vi "主函数.vi"() -> ()   [LabVIEW 2013]
uses:
  <vilib>/userdefined/High Color/IMAQdx.ctl
  <vilib>/Analysis/Matrix/Numeric/Conversions/Array To Matrix - RA2.vi
  <vilib>/Analysis/Matrix/Numeric/Conversions/Matrix To Array - RM.vi
  <vilib>/Analysis/Matrix/NI_Matrix.lvlib
  <vilib>/vision/driver/NI_Vision_Acquisition_Software.lvlib
  <vilib>/vision/NI_Vision_Development_Module.lvlib
panel:
  in  "?":enum32{"图像显示界面", "静态识别参数", "动态跟踪参数"}(tab)
  out "匹配成功":bool
  out "?":T1(plugin-control)
  in  "拍照并存储":bool
  out "系统登陆成功":bool
  in  "?":bool
  in  "模式选择":enum16{"静态人脸识别模式", "动态人脸跟踪模式", ""}(ring)=enum."动态人脸跟踪模式"
  in  "Show Templates":bool
  out "完全跟踪":bool
  in  "lower limit 2":dbl=1000.0
  in  "upper limit 2":dbl=1500000.0
  in  "上限":dbl=1500000.0
  in  "下限":dbl=1000.0
  out "半径":dbl
  in  "pen 2":T2={"Width"=1, "Style"=enum."Solid"} caption="画笔"
  out "半径 2":dbl
  out "sqrt(x)":dbl
  out "数组 1":dbl[][](array[numeric])
  out "数组 2":dbl[][](array[numeric])
  in  "fill?(F) 2":bool caption="填充？(F)"
  out "x 2":dbl=128.0
  out "y 2":dbl=84.0
  out "x":dbl=128.0
  out "y":dbl=84.0
  in  "Lip Min Score":sgl=700.0
  in  "Nose Min Score":sgl=700.0
  in  "Eye Min Score":sgl=700.0
  in  "Options":T3={"Level"=4, "maxiteration"=20, "windowsize"=20, "threshold"=1.0}
  out "Eye Template":T1(plugin-control)
  out "Nose Template":T1(plugin-control)
  out "Lips Template":T1(plugin-control)
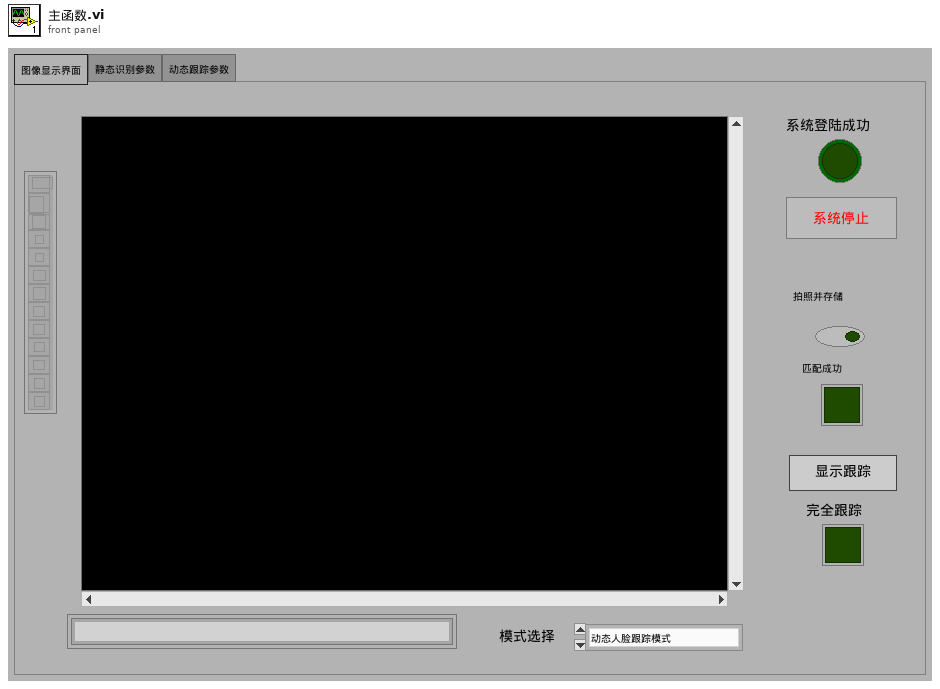
[diagram p1: front panel]
types:
  T1 = typedef "IMAQ Image.ctl" = refnum<image>
  T2 = cluster{"Width":u16, "Style":enum32{"Solid", "Dash", "Dot", "DashDot", "DashDotDot"}}
  T3 = cluster{"Level":i32, "maxiteration":i32, "windowsize":i32, "threshold":dbl}
  T4 = typedef "IMAQdx.ctl" = refnum<k21>
  T5 = typedef "Image Type" = u32
  T6 = cluster{"Position":cluster{"x":sgl, "y":sgl}, "Angle":sgl, "Scale":sgl, "Score":sgl, "Bounding Box":cluster{"x":sgl, "y":sgl}[]}[]
  T7 = typedef "imagedata.ctl" = cluster{"image type":i32, "image depth":i32, "image":u8[], "mask":u8[], "colors":u32[], "Rectangle":cluster{"left":i16, "top":i16, "right":i16, "bottom":i16}}
  T8 = cluster{"left":i16, "top":i16, "right":i16, "bottom":i16}
  T9 = typedef "NI_Matrix.lvlib/RealMatrix.ctl" = dbl[][]
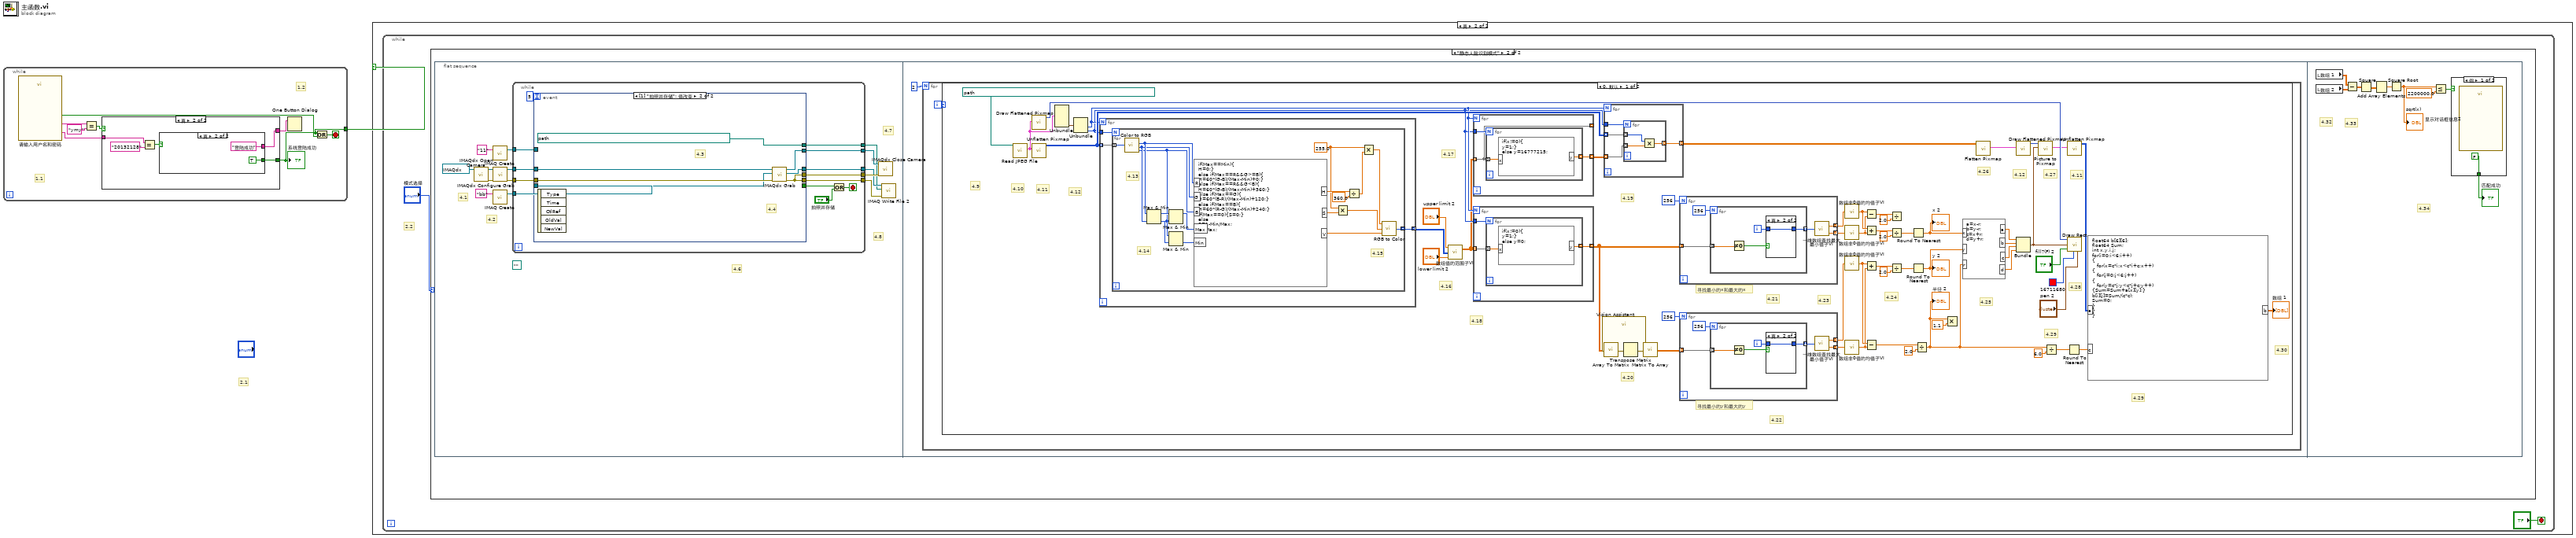
[diagram p0: block diagram]
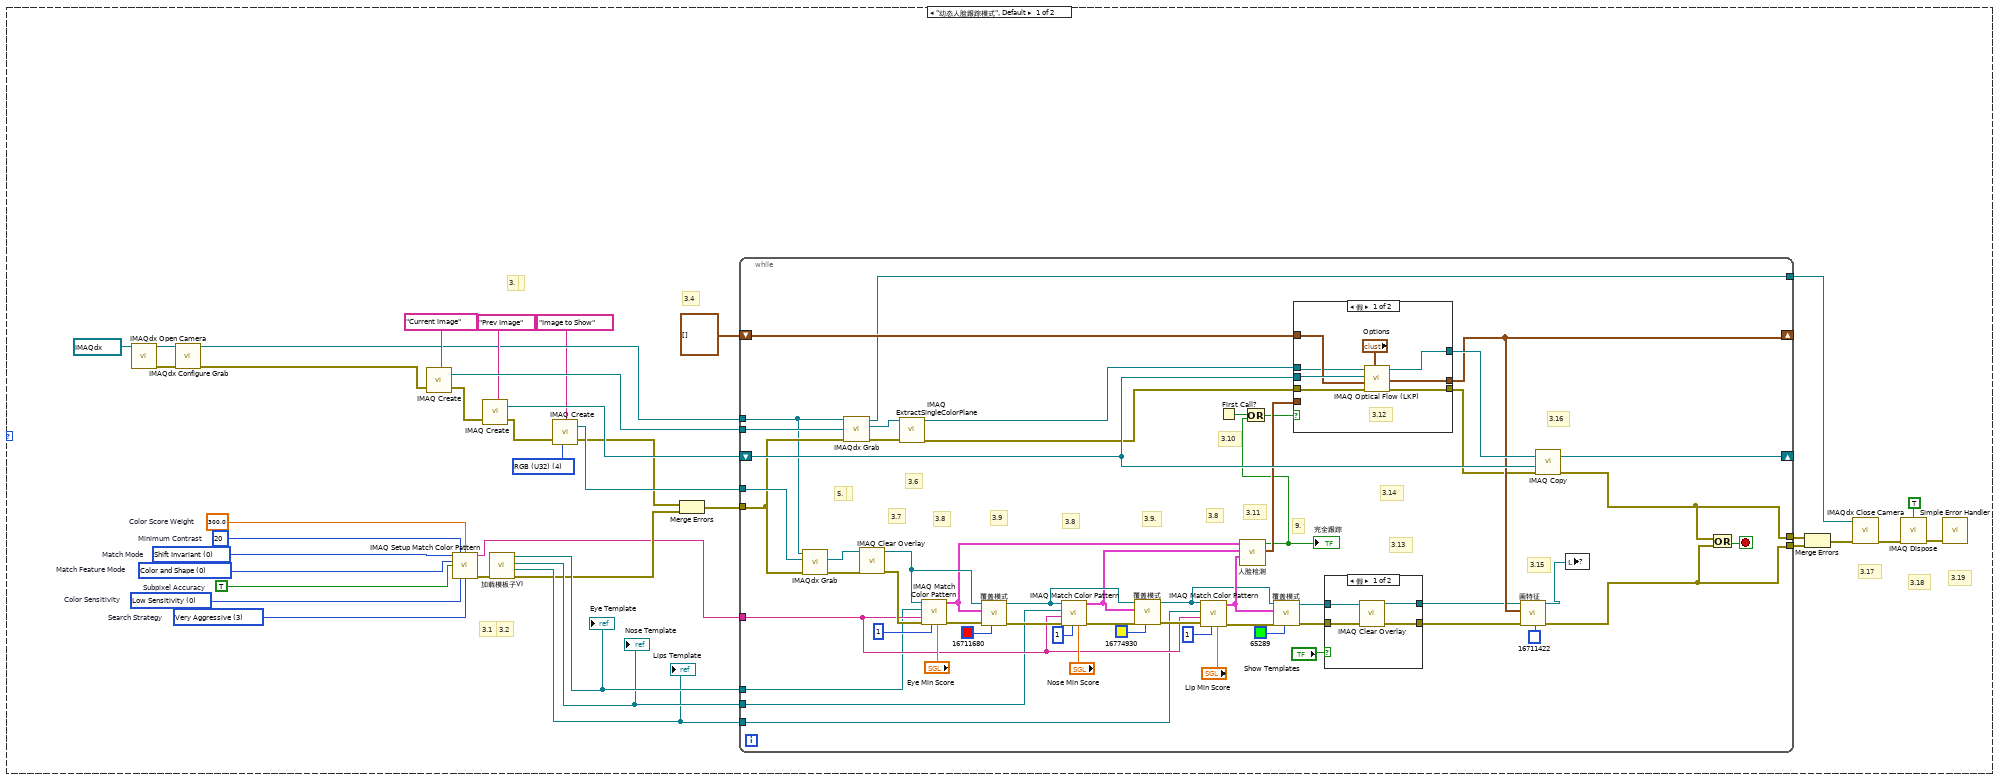
[diagram p3: hidden frame]
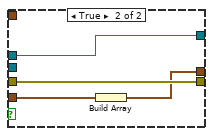
[diagram p5: hidden frame]
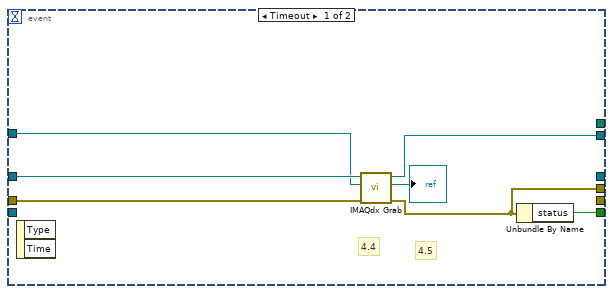
[diagram p6: hidden frame]
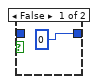
[diagram p7: hidden frame]
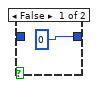
[diagram p8: hidden frame]
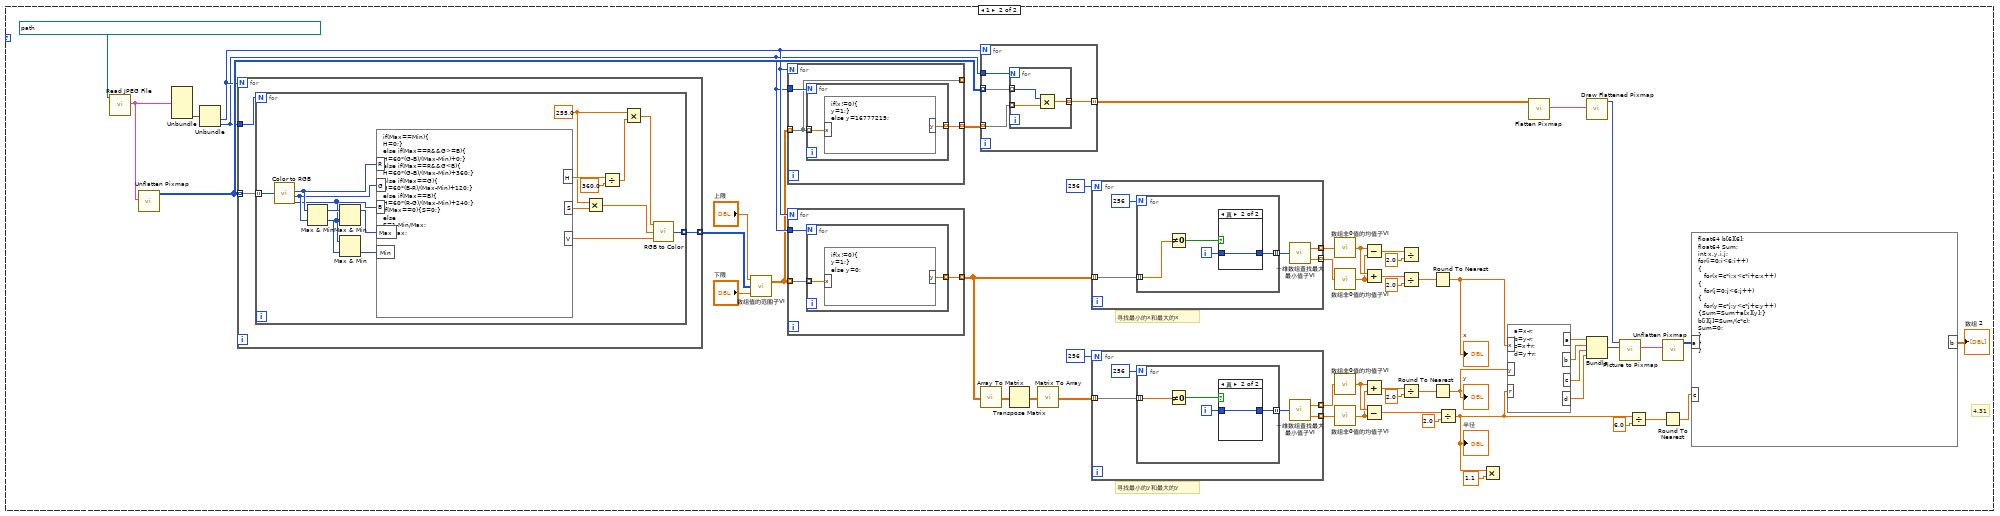
[diagram p9: hidden frame]
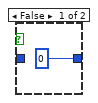
[diagram p10: hidden frame]
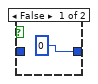
[diagram p11: hidden frame]
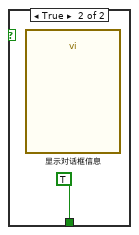
[diagram p12: hidden frame]
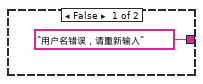
[diagram p13: hidden frame]
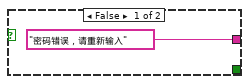
[diagram p14: hidden frame]
diagram:
  # "2.1"
  n1 = while {
    tunnel: [w2] -> w1
    stop <- w3 stop-if-true
    # "1.2"
    # "1.1"
    n2 = call "请输入用户名和密码"() -> ("密码"=w6:string, "用户名"=w8:string, "取消登陆"=w4:bool)  [unwired: 16 in, 1 out]
    n3 = Equal?(x=w8, y="ymy") -> (x = y?=w7:bool)
    n4 = case shown="真" w7 {
      tunnel: w6 -> [_ w14]
      tunnel: [_ w12] -> w2
      tunnel: ["用户名错误，请重新输入" w11] -> w5
      frame False {
      }
      frame True {
        n5 = Equal?(x=w14, y="20132128") -> (x = y?=w15:bool)
        n6 = case shown="真" w15 {
          tunnel: [_ TRUE] -> w12
          tunnel: ["密码错误，请重新输入" "登陆成功"] -> w11
          frame False {
          }
          frame True {
          }
        }
      }
    }
    "系统登陆成功" <- w2
    n7 = One Button Dialog(message=w5) -> ()  [unwired: 1 in, 1 out]
    n8 = Or(x=w2, y=w4) -> (x .or. y?=w3:bool)
  }
  n9 = case shown="真" w1 {
    frame False {
    }
    frame True {
      n10 = while {
        stop <- "?" stop-if-true
        # "2.2"
        n11 = case shown="\"静态人脸识别模式\"" "模式选择" {
          frame "动态人脸跟踪模式", Default {
            w37 = T5 4 items=["Grayscale (U8)", "Grayscale (I16)", "Grayscale (SGL)", "Complex (CSG)", "RGB (U32)", "HSL (U32)", "RGB (U64)", "Grayscale (U16)"] ("Image Type")
            w41 = TRUE  # Subpixel Accuracy
            w47 = u32 0 items=["Color and Shape", "Color", "Shape"]  # Match Feature Mode
            w46 = u32 3 items=["Conservative", "Balance", "Aggressive", "Very Aggressive"]  # Search Strategy
            w45 = 20  # Minimum Contrast
            w44 = sgl 300.0  # Color Score Weight
            w43 = u32 0 items=["Low Sensitivity", "Medium Sensitivity", "High Sensitivity"]  # Color Sensitivity
            w42 = u32 0 items=["Shift Invariant", "Rotation Invariant"]  # Match Mode
            # "3.19"
            # "3.17"
            # "3.4"
            # "3.3"
            # "3."
            # "3."
            # "3.2"
            # "3.1"
            # "3.18"
            n12 = call <vilib>:"IMAQdx Open Camera.vi"("Session In"=T4 "cam0") -> ("error out"=w51:errorcluster, "Session Out"=w52:T4)  [unwired: 9 in]
            n13 = call <vilib>:"IMAQdx Configure Grab.vi"("error in"=w51, "Session In"=w52) -> ("error out"=w30:errorcluster, "Session Out"=w48:T4)  [unwired: 8 in]
            n14 = call "IMAQ Create"("Image Name"="Current Image", "error in (no error)"=w30) -> ("New Image"=w56:T1, "error out"=w29:errorcluster)  [unwired: 2 in, 1 out]
            n15 = call "IMAQ Setup Match Color Pattern"("Match Mode"=w42, "Minimum Contrast"=w45, "Color Score Weight"=w44, "Match Feature Mode"=w47, "Subpixel Accuracy"=w41, "Color Sensitivity"=w43, "Search Strategy"=w46) -> ("Match Color Pattern Setup Data"=w24:string, "error out"=w40:errorcluster)  [unwired: 7 in]
            n16 = call "IMAQ Create"("Image Name"="Prev Image", "error in (no error)"=w29) -> ("New Image"=w49:T1, "error out"=w28:errorcluster)  [unwired: 2 in, 1 out]
            n17 = call "加载模板子VI.vi"("error in (no error)"=w40) -> ("error out"=w26:errorcluster, "Lips Template"=w34:T1, "Nose Template"=w35:T1, "Eye Template"=w36:T1)  [unwired: 7 in]
            "Eye Template" <- w36
            "Nose Template" <- w35
            "Lips Template" <- w34
            n18 = call "IMAQ Create"("Image Name"="Image to Show", "Image Type"=w37, "error in (no error)"=w28) -> ("New Image"=w38:T1, "error out"=w27:errorcluster)  [unwired: 1 in, 1 out]
            n19 = Merge Errors(w27, w26) -> (w25:errorcluster)
            n20 = while {
              tunnel: w56 -> [w110]
              shift-right: [w112] -> _
              shift-left: w49 -> [w113]
              shift-right: [w74] -> _
              shift-left: cluster{"X":sgl, "Y":sgl}[] [] ("Feature Points Out") -> [w111]
              tunnel: w48 -> [w65]
              tunnel: [w109] -> w54
              tunnel: w24 -> [w82]
              tunnel: w36 -> [w81]
              tunnel: w35 -> [w80]
              tunnel: w34 -> [w79]
              tunnel: w38 -> [w77]
              tunnel: w25 -> [w67]
              tunnel: [w63] -> w23
              tunnel: [w58] -> w22
              stop <- w64 stop-if-true
              # "3.10"
              # "3.16"
              # "3.15"
              # "3.14"
              # "3.13"
              # "3.11"
              # "9."
              # "3.8"
              # "3.9."
              # "3.8"
              # "3.9"
              # "3.8"
              # "3.7"
              # "3.6"
              # "3.5"
              # "5."
              n21 = call <vilib>:"IMAQdx Grab.vi"("error in"=w67, "Image In"=w77, "Session In"=w65) -> ("error out"=w76:errorcluster, "Image Out"=w75:T1)  [unwired: 5 in, 2 out]
              n22 = call <vilib>:"IMAQdx Grab.vi"("error in"=w67, "Image In"=w110, "Session In"=w65) -> ("error out"=w106:errorcluster, "Image Out"=w83:T1, "Session Out"=w109:T4)  [unwired: 5 in, 1 out]
              n23 = call "IMAQ Clear Overlay"("error in (no error)"=w76, "Image"=w75) -> ("error out"=w104:errorcluster, "Image Out"=w90:T1)  [unwired: 8 in]
              n24 = call "IMAQ ExtractSingleColorPlane"("error in (no error)"=w106, "Image Src"=w83) -> ("error out"=w108:errorcluster, "Image Dst Out"=w107:T1)  [unwired: 8 in]
              n25 = call "IMAQ Match Color Pattern"("Minimum Match Score"="Eye Min Score", "Number of Matches Requested"=1, "error in (no error)"=w104, "Match Color Pattern Setup Data"=w82, "Template Image"=w81, "Image"=w90) -> ("error out"=w103:errorcluster, "Matches"=w87:T6)  [unwired: 3 in, 1 out]
              n26 = call "覆盖模式.vi"("Color"=u32 16711680, "error in"=w103, "Matches"=w87, "Image"=w90) -> ("error out"=w100:errorcluster, "Image Out"=w97:T1)  [unwired: 6 in]
              n27 = call "IMAQ Match Color Pattern"("Minimum Match Score"="Nose Min Score", "Number of Matches Requested"=1, "error in (no error)"=w100, "Match Color Pattern Setup Data"=w82, "Template Image"=w80, "Image"=w97) -> ("error out"=w98:errorcluster, "Matches"=w86:T6)  [unwired: 3 in, 1 out]
              n28 = call "覆盖模式.vi"("Color"=u32 16774930, "error in"=w98, "Matches"=w86, "Image"=w97) -> ("error out"=w96:errorcluster, "Image Out"=w84:T1)  [unwired: 6 in]
              n29 = call "IMAQ Match Color Pattern"("Minimum Match Score"="Lip Min Score", "Number of Matches Requested"=1, "error in (no error)"=w96, "Match Color Pattern Setup Data"=w82, "Template Image"=w79, "Image"=w84) -> ("error out"=w95:errorcluster, "Matches"=w85:T6)  [unwired: 3 in, 1 out]
              n30 = First Call?() -> (First Call?: T/F=w60:bool)
              n31 = call "人脸检测.vi"("Lips Match"=w85, "Nose Match"=w86, "Eye Match"=w87) -> ("Lip Position"=w78:cluster{"x":sgl, "y":sgl}, "Face Found"=w62:bool)  [unwired: 6 in, 1 out]
              "完全跟踪" <- w62
              n32 = Or(x=w60, y=w62) -> (x .or. y?=w61:bool)
              n33 = call "覆盖模式.vi"("Color"=u32 65289, "error in"=w95, "Matches"=w85, "Image"=w84) -> ("error out"=w70:errorcluster, "Image Out"=w72:T1)  [unwired: 6 in]
              n34 = case shown="假" w61 {
                tunnel: w113 -> [w127 _]
                tunnel: w111 -> [w126 _]
                tunnel: [w125 w128] -> w74
                tunnel: w108 -> [w124 w131]
                tunnel: w107 -> [w120 w130]
                tunnel: [w122 w130] -> w105
                tunnel: [w121 w131] -> w66
                tunnel: w78 -> [_ w129]
                frame False {
                  # "3.12"
                  n35 = call "IMAQ Optical Flow (LKP)"("Options"="Options", "error in (no error)"=w124, "Feature Points In"=w126, "Previous Frame"=w127, "Current Frame"=w120) -> ("error out"=w121:errorcluster, "Feature Points Out"=w125:cluster{"X":sgl, "Y":sgl}[], "Current Frame Out (dup)"=w122:T1)  [unwired: 1 in, 3 out]
                }
                frame True {
                  n36 = Build Array(w129) -> (w128:cluster{"x":sgl, "y":sgl}[])
                }
              }
              n37 = case shown="假" "Show Templates" {
                tunnel: w72 -> [w117 w119]
                tunnel: [w116 w119] -> w71
                tunnel: w70 -> [w115 w118]
                tunnel: [w114 w118] -> w68
                frame False {
                  n38 = call "IMAQ Clear Overlay"("error in (no error)"=w115, "Image"=w117) -> ("error out"=w114:errorcluster, "Image Out"=w116:T1)  [unwired: 8 in]
                }
                frame True {
                }
              }
              n39 = call "画特征.vi"("Color"=u32 16711422, "Error In"=w68, "Feature Ponts"=w74, "Image"=w71) -> ("Error Out"=w58:errorcluster, "Image Out"=w59:T1)  [unwired: 6 in]
              n40 = call "IMAQ Copy"("error in (no error)"=w66, "Image Dst"=w113, "Image Src"=w105) -> ("error out"=w63:errorcluster, "Image Dst Out"=w112:T1)  [unwired: 3 out]
              n41 = local write item#18(w59) -> ()
              n42 = Compound Arithmetic op=OR(w63, w58) -> (w64:bool)
            }
            n43 = Merge Errors(w23, w22) -> (w21:errorcluster)
            n44 = call <vilib>:"IMAQdx Close Camera.vi"("error in"=w21, "Session In"=w54) -> ("error out"=w33:errorcluster)  [unwired: 9 in]
            n45 = call "IMAQ Dispose"("All Images? (No)"=TRUE, "error in (no error)"=w33) -> ("error out"=w32:errorcluster)  [unwired: 1 in, 3 out]
            n46 = call <vilib>:"Simple Error Handler.vi"("error in (no error)"=w32) -> ()  [unwired: 1 in, 8 out]
          }
          frame "静态人脸识别模式" {
            n47 = flat-sequence {
              frame #0 {
                (unwired) path ""
                # "4.8"
                # "4.7"
                # "4.2"
                # "4.1"
                # "4.6"
                n48 = call <vilib>:"IMAQdx Open Camera.vi"("Session In"=T4 "cam0") -> ("error out"=w142:errorcluster, "Session Out"=w143:T4)  [unwired: 9 in]
                n49 = call "IMAQ Create"("Image Name"="11") -> ("New Image"=w137:T1)  [unwired: 4 in, 1 out]
                n50 = call "IMAQ Create"("Image Name"="bb") -> ("New Image"=w135:T1)  [unwired: 4 in, 1 out]
                n51 = call <vilib>:"IMAQdx Configure Grab.vi"("error in"=w142, "Session In"=w143) -> ("error out"=w139:errorcluster, "Session Out"=w140:T4)  [unwired: 8 in]
                n52 = while {
                  tunnel: [w157] -> w144
                  tunnel: w139 -> [w155]
                  tunnel: w137 -> [w154]
                  tunnel: w135 -> [w153]
                  tunnel: w140 -> [w156]
                  tunnel: [w158] -> w145
                  tunnel: [w148] -> w133
                  tunnel: [w147] -> w134
                  tunnel: [w146] -> w132
                  stop <- w149 stop-if-true
                  n53 = event shown="[1] \"拍照并存储\": 值改变" {
                    selector: _ -> [_ _]
                    dyn-events: _ -> [_ _]
                    timeout: 5 -> [_ _]
                    tunnel: [w161 _] -> w150
                    tunnel: [w160 w168] -> w158
                    tunnel: [w165 w167] -> w157
                    tunnel: w156 -> [w164 w171]
                    tunnel: w155 -> [w163 w172]
                    tunnel: w154 -> [w162 _]
                    tunnel: w153 -> [_ w170]
                    tunnel: [_ w169] -> w148
                    tunnel: [_ w167] -> w147
                    tunnel: [_ path "C:/Users/yuemingyang/Desktop/虚拟仪器/Face recognition/me/me.jpg" ("File Path")] -> w146
                    event Timeout {
                      # "4.5"
                      # "4.4"
                      n54 = event-data() -> ()  [unwired: 1 in, 2 out]
                      n55 = call <vilib>:"IMAQdx Grab.vi"("error in"=w163, "Image In"=w162, "Session In"=w164) -> ("error out"=w165:errorcluster, "Image Out"=→"?":T1, "Session Out"=w160:T4)  [unwired: 5 in, 1 out]
                      n56 = Unbundle By Name(w165) -> ("status"=w161:bool)
                    }
                    event "拍照并存储": Value Change {
                      # "4.4"
                      # "4.3"
                      n57 = event-data() -> ()  [unwired: 1 in, 5 out]
                      n58 = call <vilib>:"IMAQdx Grab.vi"("error in"=w172, "Image In"=w170, "Session In"=w171) -> ("error out"=w167:errorcluster, "Image Out"=w169:T1, "Session Out"=w168:T4)  [unwired: 5 in, 1 out]
                    }
                  }
                  n59 = Or(x=w150, y="拍照并存储") -> (x .or. y?=w149:bool)
                }
                n60 = call <vilib>:"IMAQdx Close Camera.vi"("error in"=w144, "Session In"=w145) -> ()  [unwired: 9 in, 1 out]
                n61 = call-poly "IMAQ Write File 2"("error in (no error)"=w134, "File Path"=w132, "Image"=w133) -> ()  [unwired: 7 in, 2 out]
              }
              frame #1 {
                n62 = for {
                  N: 2 -> [_]
                  i -> [w174]
                  n63 = case shown="0, 默认" w174 {
                    frame 0, Default {
                      # "4.30"
                      # "4.29"
                      # "4.29"
                      # "4.28"
                      # "4.27"
                      # "4.11"
                      # "4.12"
                      # "4.26"
                      # "4.25"
                      # "4.24"
                      # "4.24"
                      # "4.24"
                      # "4.24"
                      # "4.23"
                      # "4.23"
                      # "4.22"
                      # "4.21"
                      # "4.20"
                      # "4.19"
                      # "4.18"
                      # "4.17"
                      # "4.16"
                      # "4.12"
                      # "4.11"
                      # "4.10"
                      # "4.9"
                      # "寻找最小的y和最大的y"
                      # "寻找最小的x和最大的x"
                      n64 = call <vilib>:"Read JPEG File.vi"("path to JPEG file"=path "C:/Users/yuemingyang/Desktop/虚拟仪器/Face recognition/me/me.jpg" ("File Path")) -> ("image data"=w229:T7)  [unwired: 8 in, 2 out]
                      n65 = call <vilib>:"Draw Flattened Pixmap.vi"("image data"=w229) -> ("new picture"=w198:picture)  [unwired: 8 in]
                      n66 = call <vilib>:"Unflatten Pixmap.vi"("image data"=w229) -> ("24-bit pixmap"=w201:u32[][])  [unwired: 4 in, 6 out]
                      n67 = Unbundle(w229) -> ("Rectangle"=w231:T8)  [unwired: 5 out]
                      n68 = Unbundle(w231) -> ("right"=w189:i16, "bottom"=w188:i16)  [unwired: 2 out]
                      n69 = for {
                        N: w189 -> [_]
                        tunnel: w201 -> [w273] mode=indexing
                        tunnel: [w272] -> w181 mode=indexing
                        tunnel: w188 -> [w271]
                        n70 = for {
                          N: w271 -> [_]
                          tunnel: w273 -> [w290] mode=indexing
                          tunnel: [w281] -> w272 mode=indexing
                          w286 = 255.0 ("x")
                          # "4.15"
                          # "4.14"
                          # "4.13"
                          n71 = call <vilib>:"Color to RGB.vi"("Color"=w290) -> ("R"=w276:u8, "G"=w275:u8, "B"=w274:u8)  [unwired: 1 out]
                          n72 = Max & Min(x=w276, y=w275) -> (max(x,y)=w280:u8, min(x,y)=w279:u8)
                          n73 = Max & Min(x=w280, y=w274) -> (max(x,y)=w278:u8)  [unwired: 1 out]
                          n74 = Max & Min(x=w274, y=w279) -> (min(x,y)=w277:u8)  [unwired: 1 out]
                          n75 = formula code="if(Max==Min){\nH=0;}\nelse if(Max==R&&G>=B){\nH=60*(G-B)/(Max-Min)+0;}\nelse if(Max==R&&G<B){\nH=60*(G-B)/(Max-Min)+360;}\nelse if(Max==G){\nH=60*(B-R)/(Max-Min)+120;}\nelse if(Max==B){\nH=60*(R-G)/(Max-Min)+240;}\nif(Max==0){S=0;}\nelse\nS=1-Min/Max;\nV=Max;"("R"=w276, "G"=w275, "B"=w274, "Max"=w278, "Min"=w277) -> ("H"=w288:dbl, "S"=w285:dbl, "V"=w282:dbl)
                          n76 = Multiply(x=w286, y=w285) -> (x*y=w283:dbl)
                          n77 = Divide(x=w288, y=360.0) -> (x/y=w287:dbl)
                          n78 = Multiply(x=w286, y=w287) -> (x*y=w284:dbl)
                          n79 = call <vilib>:"RGB to Color.vi"("B"=w282, "G"=w283, "R"=w284) -> ("Color"=w281:u32)
                        }
                      }
                      n80 = call "数组值的范围子VI.vi"("下限"="lower limit 2", "数组"=w181, "上限"="upper limit 2") -> ("数组 2"=w180:dbl[][])  [unwired: 2 in]
                      n81 = for {
                        N: w189 -> [_]
                        tunnel: w188 -> [w234]
                        tunnel: [w232] -> _ mode=indexing
                        tunnel: [w233] -> w202 mode=indexing
                        tunnel: w180 -> [w232] mode=indexing
                        n82 = for {
                          N: w234 -> [_]
                          tunnel: w232 -> [w236] mode=indexing
                          tunnel: [w235] -> w233 mode=indexing
                          n83 = formula code="if(x!=0){\ny=1;}\nelse y=16777215;"("x"=w236) -> ("y"=w235:dbl)
                        }
                      }
                      n84 = for {
                        N: w189 -> [_]
                        tunnel: w188 -> [w268]
                        tunnel: w180 -> [w267] mode=indexing
                        tunnel: [w266] -> w204 mode=indexing
                        n85 = for {
                          N: w268 -> [_]
                          tunnel: w267 -> [w270] mode=indexing
                          tunnel: [w269] -> w266 mode=indexing
                          n86 = formula code="if(x!=0){\ny=1;}\nelse y=0;"("x"=w270) -> ("y"=w269:dbl)
                        }
                      }
                      n87 = call "Vision Assistant"() -> ()  [unwired: 12 in]
                      n88 = for {
                        N: w189 -> [_]
                        tunnel: w188 -> [w262]
                        tunnel: w202 -> [w261] mode=indexing
                        tunnel: w201 -> [w260] mode=indexing
                        tunnel: [w259] -> w228 mode=indexing
                        n89 = for {
                          N: w262 -> [_]
                          tunnel: w261 -> [w265] mode=indexing
                          tunnel: w260 -> [w264] mode=indexing
                          tunnel: [w263] -> w259 mode=indexing
                          n90 = Multiply(x=w264, y=w265) -> (x*y=w263:dbl)
                        }
                      }
                      n91 = call-poly <vilib>:"Array To Matrix.vi"("Real 2D Array"=w204) -> ("Real Matrix"=w224:T9)
                      n92 = Transpose Matrix(1:w224) -> (0:w223:T9)
                      n93 = call-poly <vilib>:"Matrix To Array.vi"("Real Matrix"=w223) -> ("Real 2D Array"=w218:dbl[][])
                      n94 = for {
                        N: 256 -> [_]
                        tunnel: w204 -> [w251] mode=indexing
                        tunnel: [w249] -> w216 mode=indexing
                        tunnel: [w248] -> w215 mode=indexing
                        n95 = for {
                          N: 256 -> [_]
                          tunnel: w251 -> [w255] mode=indexing
                          tunnel: [w253] -> w250 mode=indexing
                          i -> [w254]
                          n96 = Not Equal To 0?(x=w255) -> (x != 0?=w256:bool)
                          n97 = case shown="真" w256 {
                            tunnel: [0 w258] -> w253
                            tunnel: w254 -> [_ w258]
                            frame False {
                            }
                            frame True {
                            }
                          }
                        }
                        n98 = call "一维数组查找最大最小值子VI.vi"("数组 3"=w250) -> ("最小值"=w248:dbl, "最大值"=w249:dbl)  [unwired: 2 in]
                      }
                      n99 = for {
                        N: 256 -> [_]
                        tunnel: w218 -> [w240] mode=indexing
                        tunnel: [w238] -> w214 mode=indexing
                        tunnel: [w237] -> w213 mode=indexing
                        n100 = for {
                          N: 256 -> [_]
                          tunnel: w240 -> [w244] mode=indexing
                          tunnel: [w242] -> w239 mode=indexing
                          i -> [w243]
                          n101 = Not Equal To 0?(x=w244) -> (x != 0?=w245:bool)
                          n102 = case shown="真" w245 {
                            tunnel: [0 w247] -> w242
                            tunnel: w243 -> [_ w247]
                            frame False {
                            }
                            frame True {
                            }
                          }
                        }
                        n103 = call "一维数组查找最大最小值子VI.vi"("数组 3"=w239) -> ("最小值"=w237:dbl, "最大值"=w238:dbl)  [unwired: 2 in]
                      }
                      n104 = call "数组非0值的均值子VI.vi"("数组"=w216) -> ("平均值"=w210:dbl)  [unwired: 2 in]
                      n105 = call "数组非0值的均值子VI.vi"("数组"=w215) -> ("平均值"=w209:dbl)  [unwired: 2 in]
                      n106 = call "数组非0值的均值子VI.vi"("数组"=w214) -> ("平均值"=w206:dbl)  [unwired: 2 in]
                      n107 = call "数组非0值的均值子VI.vi"("数组"=w213) -> ("平均值"=w205:dbl)  [unwired: 2 in]
                      n108 = Subtract(x=w210, y=w209) -> (x-y=w212:dbl)
                      n109 = Add(x=w210, y=w209) -> (x+y=w217:dbl)
                      n110 = Add(x=w206, y=w205) -> (x+y=w221:dbl)
                      n111 = Subtract(x=w206, y=w205) -> (x-y=w208:dbl)
                      n112 = Divide(x=w212, y=2.0) -> ()  [unwired: 1 out]
                      n113 = Divide(x=w217, y=2.0) -> (x/y=w225:dbl)
                      n114 = Divide(x=w221, y=2.0) -> (x/y=w219:dbl)
                      n115 = Round To Nearest(number=w225) -> (nearest integer value=w197:dbl)
                      "x 2" <- w197
                      n116 = Round To Nearest(number=w219) -> (nearest integer value=w196:dbl)
                      "y 2" <- w196
                      n117 = Divide(x=w208, y=2.0) -> (x/y=w178:dbl)
                      "半径 2" <- w178
                      n118 = Multiply(x=w178, y=1.1) -> ()  [unwired: 1 out]
                      n119 = formula code="a=x-r;\nb=y-r;\nc=x+r;\nd=y+r;"("x"=w197, "y"=w196, "r"=w178) -> ("a"=w195:dbl, "b"=w194:dbl, "c"=w193:dbl, "d"=w192:dbl)
                      n120 = call <vilib>:"Flatten Pixmap.vi"("24-bit pixmap"=w228) -> ("image data"=w230:T7)  [unwired: 10 in]
                      n121 = call <vilib>:"Draw Flattened Pixmap.vi"("image data"=w230) -> ("new picture"=w190:picture)  [unwired: 8 in]
                      n122 = Bundle("a"=w195, "b"=w194, "c"=w193, "d"=w192) -> (w191:cluster{"a":dbl, "b":dbl, "c":dbl, "d":dbl})  [unwired: 1 in]
                      n123 = call <vilib>:"Picture to Pixmap.vi"("rect"=w191, "picture"=w190) -> ("image data"=w187:T7)  [unwired: 8 in, 1 out]
                      n124 = Divide(x=w178, y=6.0) -> (x/y=w177:dbl)
                      n125 = Round To Nearest(number=w177) -> (nearest integer value=w176:dbl)
                      n126 = call <vilib>:"Unflatten Pixmap.vi"("image data"=w187) -> ("24-bit pixmap"=w186:u32[][])  [unwired: 4 in, 6 out]
                      n127 = call <vilib>:"Draw Rect.vi"("picture"=w198, "rect"=w191, "fill?(F)"="fill?(F) 2", "color(black)"=u32 16711680, "pen"="pen 2") -> ()  [unwired: 4 in, 1 out]
                      n128 = formula code="float64 b[6][6];\nfloat64 Sum;\nint x,y,i,j;\nfor(i=0;i<6;i++)\n{\n   for(x=c*i;x<c*i+c;x++)\n{\n   for(j=0;j<6;j++)\n{\n   for(y=c*j;y<c*j+c;y++)\n{Sum=Sum+a[x][y];}\nb[i][j]=Sum/(c*c);\nSum=0;\n}\n}\n}"("a"=w186, "c"=w176) -> ("b"=→"数组 1":dbl[][])
                    }
                    frame 1 {
                      # "4.31"
                      # "寻找最小的y和最大的y"
                      # "寻找最小的x和最大的x"
                      n129 = call <vilib>:"Read JPEG File.vi"("path to JPEG file"=path "C:/Users/yuemingyang/Desktop/虚拟仪器/Face recognition/me/storage.jpg" ("File Path")) -> ("image data"=w341:T7)  [unwired: 8 in, 2 out]
                      n130 = call <vilib>:"Unflatten Pixmap.vi"("image data"=w341) -> ("24-bit pixmap"=w313:u32[][])  [unwired: 4 in, 6 out]
                      n131 = Unbundle(w341) -> ("Rectangle"=w343:T8)  [unwired: 5 out]
                      n132 = Unbundle(w343) -> ("right"=w304:i16, "bottom"=w303:i16)  [unwired: 2 out]
                      n133 = for {
                        N: w304 -> [_]
                        tunnel: w313 -> [w385] mode=indexing
                        tunnel: [w384] -> w297 mode=indexing
                        tunnel: w303 -> [w383]
                        n134 = for {
                          N: w383 -> [_]
                          tunnel: w385 -> [w402] mode=indexing
                          tunnel: [w393] -> w384 mode=indexing
                          w398 = 255.0 ("x")
                          n135 = call <vilib>:"Color to RGB.vi"("Color"=w402) -> ("R"=w388:u8, "G"=w387:u8, "B"=w386:u8)  [unwired: 1 out]
                          n136 = Max & Min(x=w388, y=w387) -> (max(x,y)=w392:u8, min(x,y)=w391:u8)
                          n137 = Max & Min(x=w392, y=w386) -> (max(x,y)=w390:u8)  [unwired: 1 out]
                          n138 = Max & Min(x=w386, y=w391) -> (min(x,y)=w389:u8)  [unwired: 1 out]
                          n139 = formula code="if(Max==Min){\nH=0;}\nelse if(Max==R&&G>=B){\nH=60*(G-B)/(Max-Min)+0;}\nelse if(Max==R&&G<B){\nH=60*(G-B)/(Max-Min)+360;}\nelse if(Max==G){\nH=60*(B-R)/(Max-Min)+120;}\nelse if(Max==B){\nH=60*(R-G)/(Max-Min)+240;}\nif(Max==0){S=0;}\nelse\nS=1-Min/Max;\nV=Max;"("R"=w388, "G"=w387, "B"=w386, "Max"=w390, "Min"=w389) -> ("H"=w400:dbl, "S"=w397:dbl, "V"=w394:dbl)
                          n140 = Multiply(x=w398, y=w397) -> (x*y=w395:dbl)
                          n141 = Divide(x=w400, y=360.0) -> (x/y=w399:dbl)
                          n142 = Multiply(x=w398, y=w399) -> (x*y=w396:dbl)
                          n143 = call <vilib>:"RGB to Color.vi"("B"=w394, "G"=w395, "R"=w396) -> ("Color"=w393:u32)
                        }
                      }
                      n144 = call "数组值的范围子VI.vi"("下限"="下限", "数组"=w297, "上限"="上限") -> ("数组 2"=w296:dbl[][])  [unwired: 2 in]
                      n145 = for {
                        N: w304 -> [_]
                        tunnel: w303 -> [w346]
                        tunnel: [w344] -> _ mode=indexing
                        tunnel: [w345] -> w314 mode=indexing
                        tunnel: w296 -> [w344] mode=indexing
                        n146 = for {
                          N: w346 -> [_]
                          tunnel: w344 -> [w348] mode=indexing
                          tunnel: [w347] -> w345 mode=indexing
                          n147 = formula code="if(x!=0){\ny=1;}\nelse y=16777215;"("x"=w348) -> ("y"=w347:dbl)
                        }
                      }
                      n148 = for {
                        N: w304 -> [_]
                        tunnel: w303 -> [w380]
                        tunnel: w296 -> [w379] mode=indexing
                        tunnel: [w378] -> w316 mode=indexing
                        n149 = for {
                          N: w380 -> [_]
                          tunnel: w379 -> [w382] mode=indexing
                          tunnel: [w381] -> w378 mode=indexing
                          n150 = formula code="if(x!=0){\ny=1;}\nelse y=0;"("x"=w382) -> ("y"=w381:dbl)
                        }
                      }
                      n151 = for {
                        N: w304 -> [_]
                        tunnel: w303 -> [w374]
                        tunnel: w314 -> [w373] mode=indexing
                        tunnel: w313 -> [w372] mode=indexing
                        tunnel: [w371] -> w340 mode=indexing
                        n152 = for {
                          N: w374 -> [_]
                          tunnel: w373 -> [w377] mode=indexing
                          tunnel: w372 -> [w376] mode=indexing
                          tunnel: [w375] -> w371 mode=indexing
                          n153 = Multiply(x=w376, y=w377) -> (x*y=w375:dbl)
                        }
                      }
                      n154 = call-poly <vilib>:"Array To Matrix.vi"("Real 2D Array"=w316) -> ("Real Matrix"=w336:T9)
                      n155 = Transpose Matrix(1:w336) -> (0:w335:T9)
                      n156 = call-poly <vilib>:"Matrix To Array.vi"("Real Matrix"=w335) -> ("Real 2D Array"=w330:dbl[][])
                      n157 = for {
                        N: 256 -> [_]
                        tunnel: w316 -> [w363] mode=indexing
                        tunnel: [w361] -> w328 mode=indexing
                        tunnel: [w360] -> w327 mode=indexing
                        n158 = for {
                          N: 256 -> [_]
                          tunnel: w363 -> [w367] mode=indexing
                          tunnel: [w365] -> w362 mode=indexing
                          i -> [w366]
                          n159 = Not Equal To 0?(x=w367) -> (x != 0?=w368:bool)
                          n160 = case shown="真" w368 {
                            tunnel: [0 w370] -> w365
                            tunnel: w366 -> [_ w370]
                            frame False {
                            }
                            frame True {
                            }
                          }
                        }
                        n161 = call "一维数组查找最大最小值子VI.vi"("数组 3"=w362) -> ("最小值"=w360:dbl, "最大值"=w361:dbl)  [unwired: 2 in]
                      }
                      n162 = for {
                        N: 256 -> [_]
                        tunnel: w330 -> [w352] mode=indexing
                        tunnel: [w350] -> w326 mode=indexing
                        tunnel: [w349] -> w325 mode=indexing
                        n163 = for {
                          N: 256 -> [_]
                          tunnel: w352 -> [w356] mode=indexing
                          tunnel: [w354] -> w351 mode=indexing
                          i -> [w355]
                          n164 = Not Equal To 0?(x=w356) -> (x != 0?=w357:bool)
                          n165 = case shown="真" w357 {
                            tunnel: [0 w359] -> w354
                            tunnel: w355 -> [_ w359]
                            frame False {
                            }
                            frame True {
                            }
                          }
                        }
                        n166 = call "一维数组查找最大最小值子VI.vi"("数组 3"=w351) -> ("最小值"=w349:dbl, "最大值"=w350:dbl)  [unwired: 2 in]
                      }
                      n167 = call "数组非0值的均值子VI.vi"("数组"=w328) -> ("平均值"=w322:dbl)  [unwired: 2 in]
                      n168 = call "数组非0值的均值子VI.vi"("数组"=w327) -> ("平均值"=w321:dbl)  [unwired: 2 in]
                      n169 = call "数组非0值的均值子VI.vi"("数组"=w326) -> ("平均值"=w318:dbl)  [unwired: 2 in]
                      n170 = call "数组非0值的均值子VI.vi"("数组"=w325) -> ("平均值"=w317:dbl)  [unwired: 2 in]
                      n171 = Subtract(x=w322, y=w321) -> (x-y=w324:dbl)
                      n172 = Add(x=w322, y=w321) -> (x+y=w329:dbl)
                      n173 = Add(x=w318, y=w317) -> (x+y=w333:dbl)
                      n174 = Subtract(x=w318, y=w317) -> (x-y=w320:dbl)
                      n175 = Divide(x=w324, y=2.0) -> ()  [unwired: 1 out]
                      n176 = Divide(x=w329, y=2.0) -> (x/y=w337:dbl)
                      n177 = Divide(x=w333, y=2.0) -> (x/y=w331:dbl)
                      n178 = Round To Nearest(number=w337) -> (nearest integer value=w312:dbl)
                      "x" <- w312
                      n179 = Round To Nearest(number=w331) -> (nearest integer value=w311:dbl)
                      "y" <- w311
                      n180 = Divide(x=w320, y=2.0) -> (x/y=w294:dbl)
                      "半径" <- w294
                      n181 = Multiply(x=w294, y=1.1) -> ()  [unwired: 1 out]
                      n182 = formula code="a=x-r;\nb=y-r;\nc=x+r;\nd=y+r;"("x"=w312, "y"=w311, "r"=w294) -> ("a"=w310:dbl, "b"=w309:dbl, "c"=w308:dbl, "d"=w307:dbl)
                      n183 = call <vilib>:"Flatten Pixmap.vi"("24-bit pixmap"=w340) -> ("image data"=w342:T7)  [unwired: 10 in]
                      n184 = call <vilib>:"Draw Flattened Pixmap.vi"("image data"=w342) -> ("new picture"=w305:picture)  [unwired: 8 in]
                      n185 = Bundle("a"=w310, "b"=w309, "c"=w308, "d"=w307) -> (w306:cluster{"a":dbl, "b":dbl, "c":dbl, "d":dbl})  [unwired: 1 in]
                      n186 = call <vilib>:"Picture to Pixmap.vi"("rect"=w306, "picture"=w305) -> ("image data"=w302:T7)  [unwired: 8 in, 1 out]
                      n187 = Divide(x=w294, y=6.0) -> (x/y=w293:dbl)
                      n188 = Round To Nearest(number=w293) -> (nearest integer value=w292:dbl)
                      n189 = call <vilib>:"Unflatten Pixmap.vi"("image data"=w302) -> ("24-bit pixmap"=w301:u32[][])  [unwired: 4 in, 6 out]
                      n190 = formula code="float64 b[6][6];\nfloat64 Sum;\nint x,y,i,j;\nfor(i=0;i<6;i++)\n{\n   for(x=c*i;x<c*i+c;x++)\n{\n   for(j=0;j<6;j++)\n{\n   for(y=c*j;y<c*j+c;y++)\n{Sum=Sum+a[x][y];}\nb[i][j]=Sum/(c*c);\nSum=0;\n}\n}\n}"("a"=w301, "c"=w292) -> ("b"=→"数组 2":dbl[][])
                    }
                  }
                }
              }
              frame #2 {
                # "4.34"
                # "4.33"
                # "4.32"
                n191 = local read "数组 1"() -> (w411:dbl[][])
                n192 = local read "数组 2"() -> (w410:dbl[][])
                n193 = Subtract(x=w411, y=w410) -> (x-y=w409:dbl[][])
                n194 = Square(x=w409) -> (x^2=w408:dbl[][])
                n195 = Add Array Elements(numeric array=w408) -> (sum=w407:dbl)
                n196 = Square Root(x=w407) -> (sqrt(x)=w405:dbl)
                "sqrt(x)" <- w405
                n197 = Less Or Equal?(x=w405, y=2200000.0) -> (x <= y?=w404:bool)
                n198 = case shown="假" w404 {
                  tunnel: [FALSE TRUE] -> w403
                  frame False {
                    n199 = call "显示对话框信息2"() -> ()  [unwired: 10 in, 2 out]
                  }
                  frame True {
                    n200 = call "显示对话框信息"() -> ()  [unwired: 10 in, 2 out]
                  }
                }
                "匹配成功" <- w403
              }
            }
          }
        }
      }
    }
  }
